vi "9219-9237_3-2.vi"() -> ()   [LabVIEW 2013]
uses:
  <vilib>/Analysis/baseanly.llb/Mean (DBL).vi
  <vilib>/DAQmx/read.llb/DAQmx Read (Analog 1D Wfm NChan NSamp).vi
  <vilib>/measure/mascope.llb/Amplitude and Levels 1 chan.vi
  <vilib>/measure/mamon.llb/Trigger Detection for 1 Channel.vi
  <vilib>/Waveform/WDTOps.llb/WDT Append Waveforms DBL.vi
  <vilib>/DAQmx/miscellaneous.llb/DAQmx Fill In Error Info.vi
  <vilib>/measure/NI_MAPro.lvlib
  <vilib>/measure/mascope.llb/Pulse Measurements 1 chan.vi
  <vilib>/Analysis/NI_AALBase.lvlib
panel:
  in  "탭 컨트롤":T1(tab)
  in  "Force cal val":bool
  out "diff 4":dbl
  out "diff 3":dbl
  out "diff 2":dbl
  out "B 2-4":dbl(slide)
  out "B 1-3":dbl(slide)
  out "Balance 2/4":dbl format="%#_3g"
  out "Balance 1/3":dbl format="%#_3f"
  out "Triggered Force graph":waveform(dbl)(graph)
  out "bonding force":dbl caption="Bonding force (kg)" format="%0.2f"
  out "vaccum":waveform(dbl)(graph)
  out "Bondtime":dbl caption="Bonding time" format="%.3f"
  out "vacum":dbl format="%#_3f"
  out "trigger location":dbl caption="트리거 rising" format="%#.3f"
  out "trigger location 2":dbl caption="트리거 falling" format="%#.3f"
  out "level1 4":dbl caption="right F" format="%.2g"
  out "level1 3":dbl caption="rear F" format="%.2g"
  out "level1 2":dbl caption="left F" format="%.2g"
  out "level1":dbl caption="front F" format="%.2g"
  out "diff 1":dbl
  out "vaccum 차트 3":waveform(dbl)(graph)
  out "Force raw chart":waveform(dbl)[](graph)
  out "x-y 2":u32
  out "x-y":u32
  out "Filtered force 차트":waveform(dbl)[](graph)
  out "Force raw graph":waveform(dbl)[](graph)
  out "Filtered force 그래프":waveform(dbl)[](graph)
  in  "display":bool
  out "Strain front":dbl(graph)
  out "Strain left":dbl(graph)
  out "Strain rear":dbl(graph)
  out "Strain right":dbl(graph)
  out "data":dynamicdata(graph) caption="데이터"
  in  "reference levels":T2={"high ref level"=90.0, "mid ref level"=50.0, "low ref level"=10.0, "ref units"=1} caption="참조 레벨" {"ref units" items=["절대적인", "퍼센트"]; "high ref level" format="%0.2f"; "low ref level" format="%0.2f"; "mid ref level" format="%0.2f"}
  in  "percent level settings":T3={"method"=enum."auto select", "histogram size"=256, "histogram method"=enum."mode", "reserved"=1.0} caption="퍼센트 레벨 셋팅" {"reserved" format="%0.2f"}
  in  "bonding time trigger edge level":dbl=0.2 format="%#_13g"
  out "front mean":dbl format="%0.2f"
  out "left mean":dbl format="%0.2f"
  out "rear mean 3":dbl format="%0.2f"
  out "right mean 4":dbl format="%0.2f"
  in  "Force trigger minimum level":dbl=0.5 format="%#_13g"
  out "force offset":dbl
  in  "정지":bool
  # "Die Attach Machine Monitoring"
  # "1> 앞쪽 힘이 큰 경우\n1< 뒷쪽 힘이 큰 경우"
  # "1> 왼쪽 힘이 큰 경우\n1< 오른쪽 힘이 큰 경우"
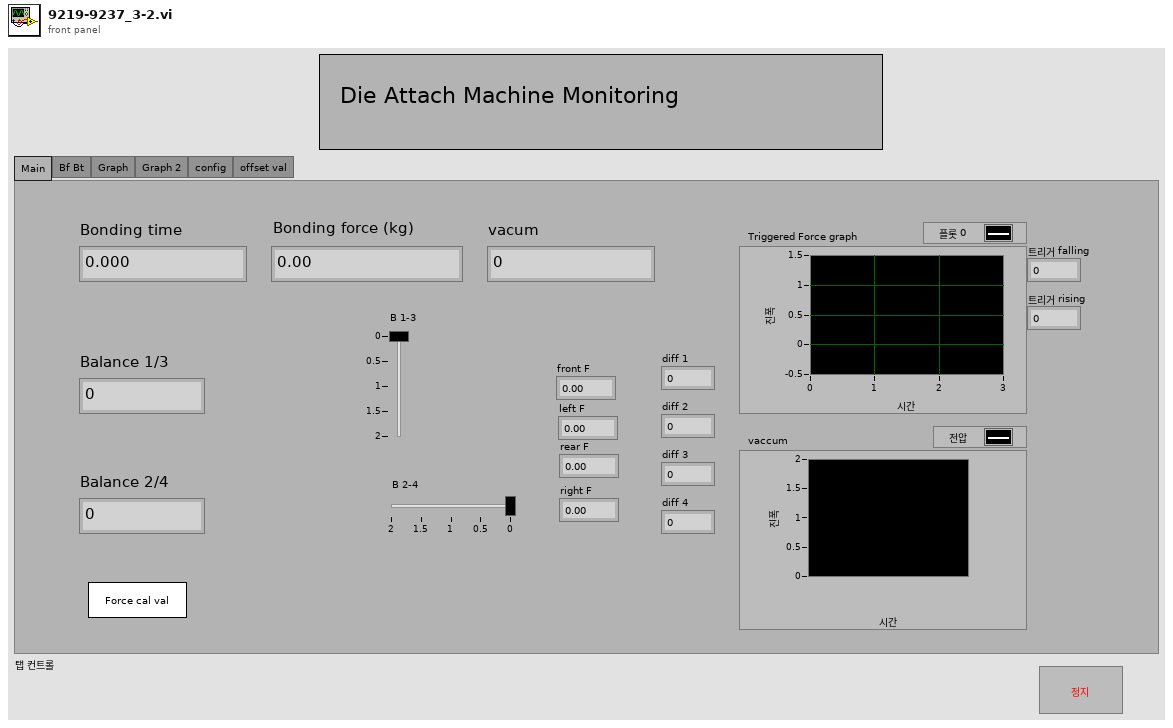
[diagram p1: front panel]
types:
  T1 = enum32{"Main", "Bf Bt", "Graph", "Graph 2", "config", "offset val"}
  T2 = cluster{"high ref level":dbl, "mid ref level":dbl, "low ref level":dbl, "ref units":u16}
  T3 = cluster{"method":enum32{"histogram", "peak", "auto select"}, "histogram size":i32, "histogram method":enum16{"mode"}, "reserved":dbl}
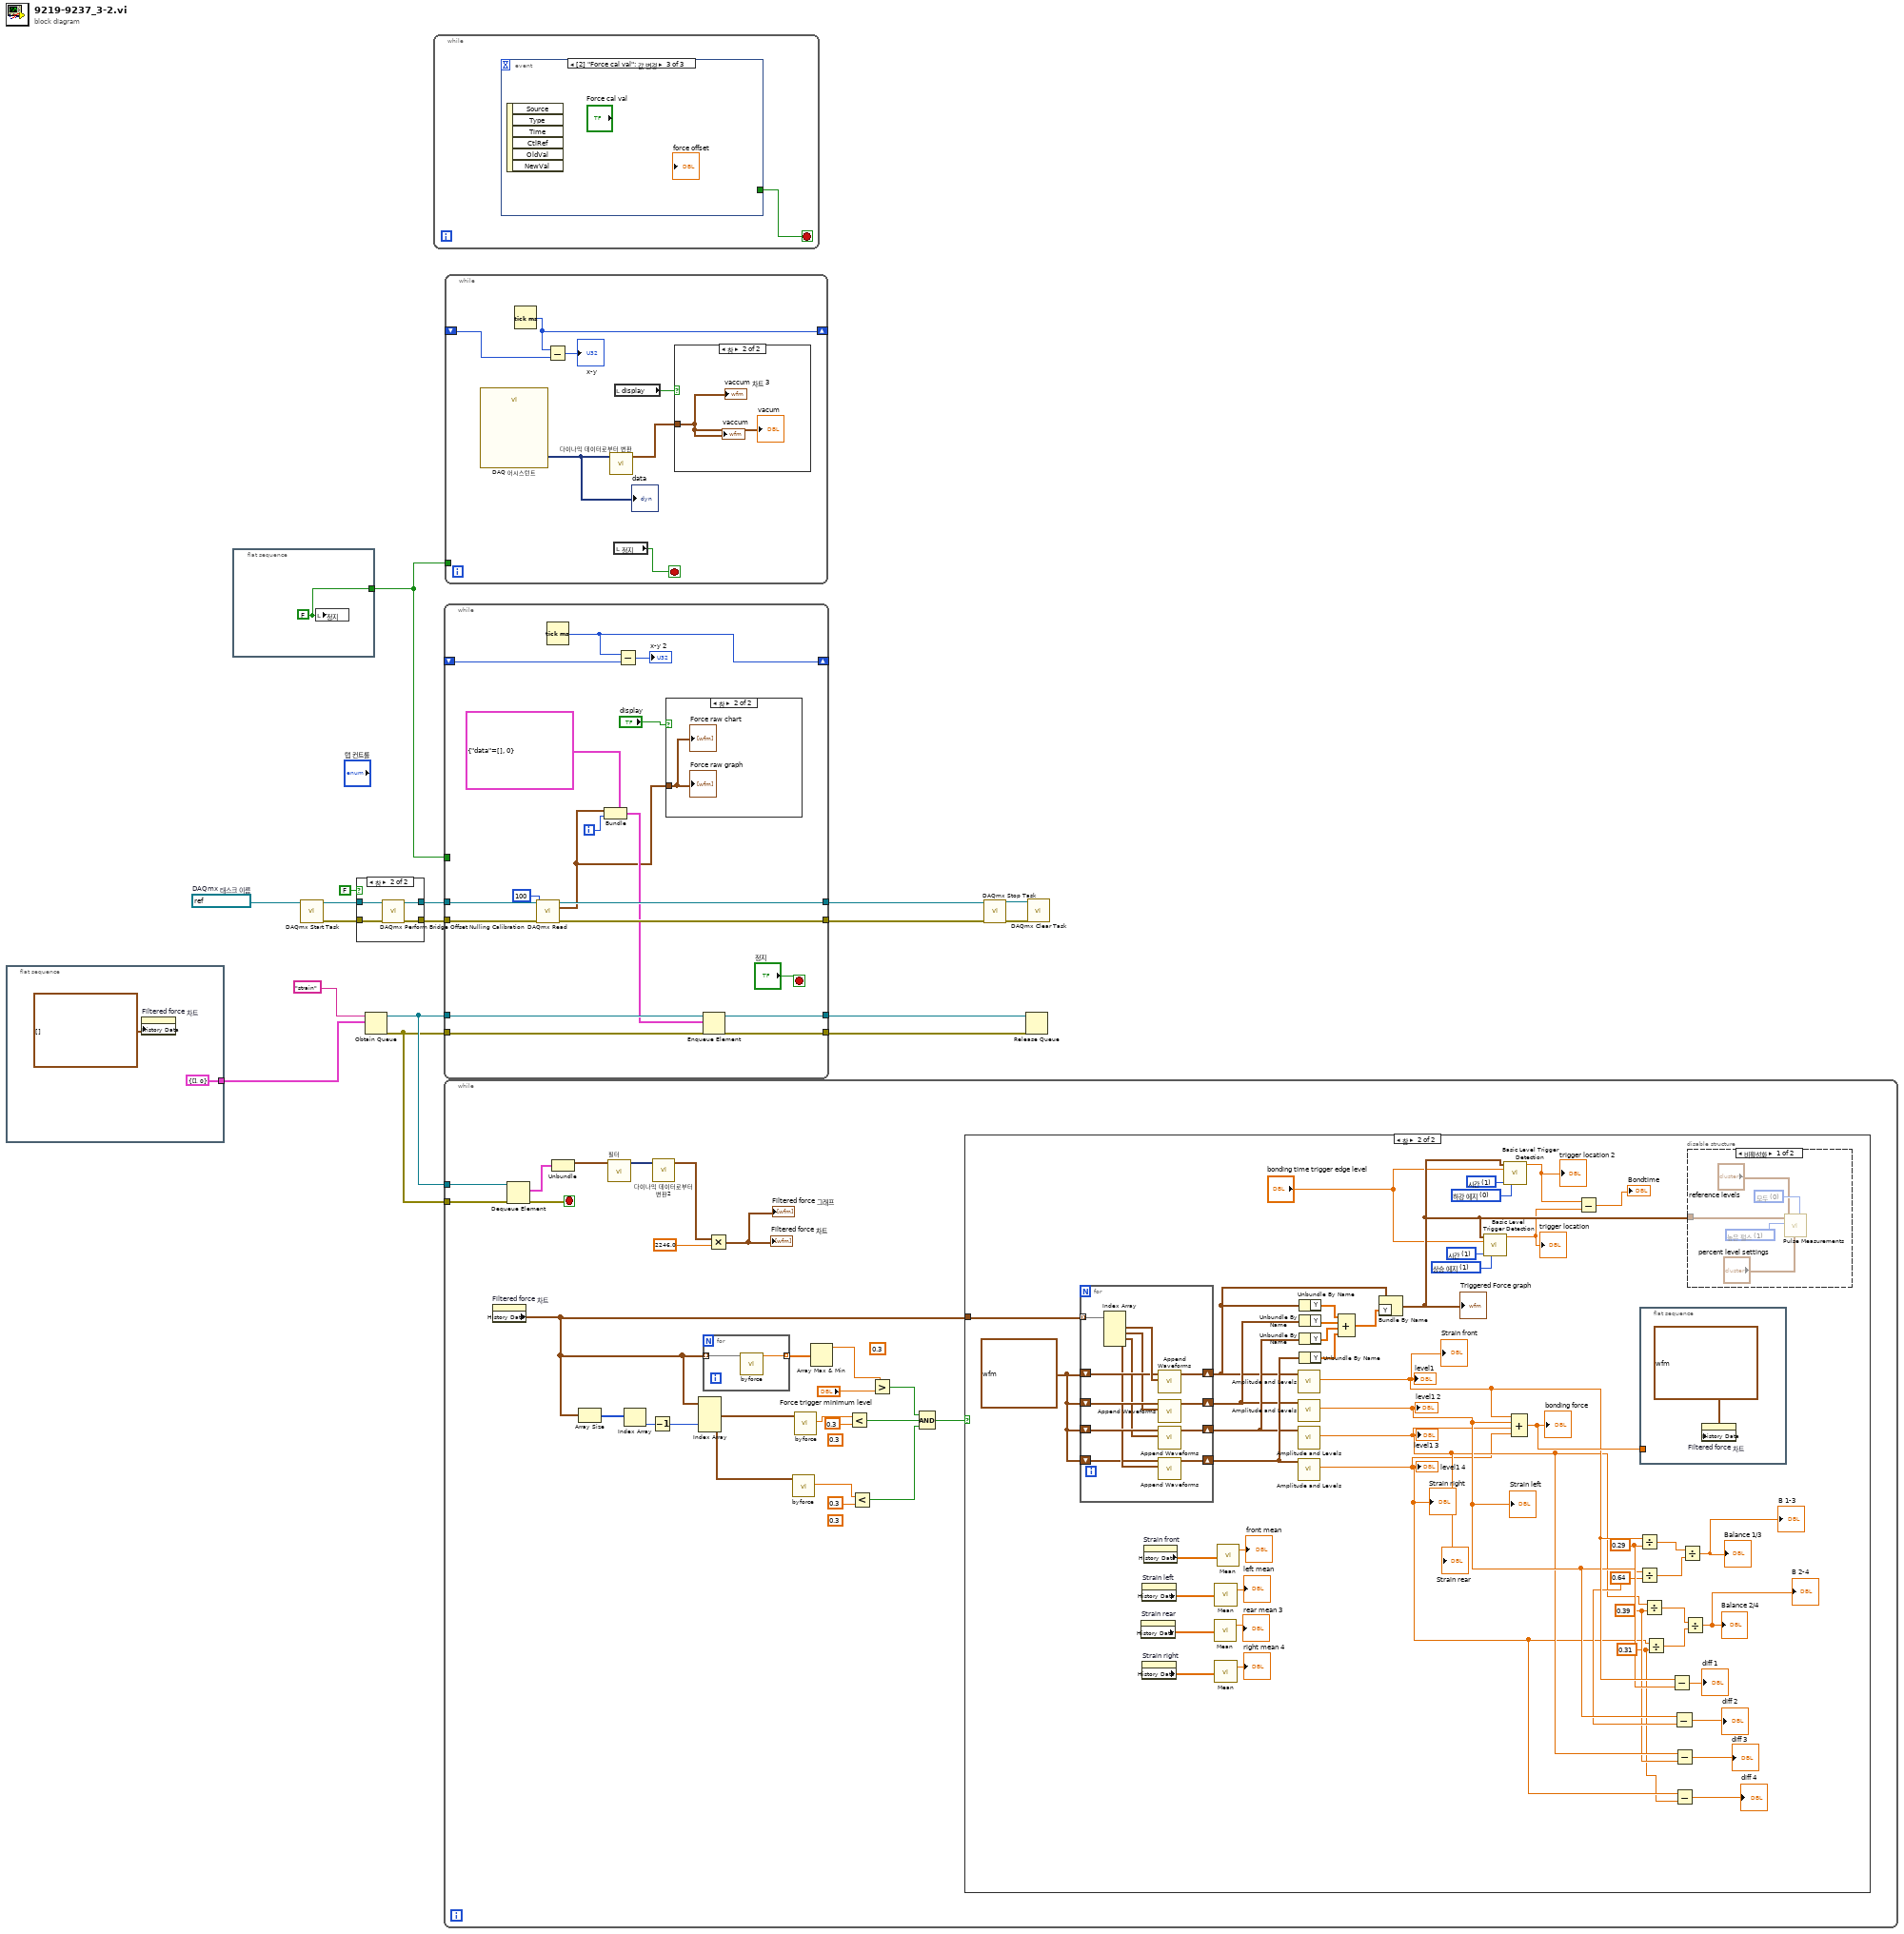
[diagram p0: block diagram]
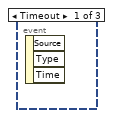
[diagram p3: hidden frame]
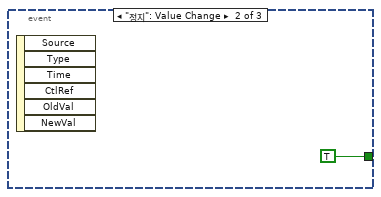
[diagram p4: hidden frame]
diagram:
  w15 = refnum<k21> "9237_task"  # DAQmx 태스크 이름
  n1 = flat-sequence {
    tunnel: [cluster{"data":waveform(dbl)[], i32} {"data"=[], 0}] -> w6
    frame #0 {
      n2 = property on="Filtered force 차트" class="WFChart (엄격한)"("History Data"=waveform(dbl)[][] [] ("히스토리 데이터")) -> ()  [unwired: 2 in, 2 out]
    }
  }
  n3 = flat-sequence {
    tunnel: [w20] -> w12
    frame #0 {
      w20 = FALSE ("정지")
      n4 = local write "정지"(w20) -> ()
    }
  }
  n5 = call <vilib>:"DAQmx Start Task.vi"("task/channels in"=w15) -> ("task out"=w5:refnum<k21>, "error out"=w4:errorcluster)  [unwired: 13 in]
  n6 = case shown="참" FALSE {
    tunnel: w5 -> [w22 w26]
    tunnel: w4 -> [w21 w25]
    tunnel: [w21 w24] -> w3
    tunnel: [w22 w23] -> w2
    frame False {
    }
    frame True {
      n7 = call <vilib>:"DAQmx Perform Bridge Offset Nulling Calibration.vi"("task/channels in"=w26, "error in"=w25) -> ("task out"=w23:refnum<k21>, "error out"=w24:errorcluster)  [unwired: 12 in]
    }
  }
  n8 = Obtain Queue(name (unnamed)="strain" ("이름(이름없음)"), element data type=w6) -> (queue out=w10:refnum<queue>, error out=w8:errorcluster)  [unwired: 3 in, 1 out]
  n9 = while {
    stop <- w27 stop-if-true
    n10 = event shown="[2] \"Force cal val\": 값 변경" {
      selector: _ -> [_ _ _]
      dyn-events: _ -> [_ _ _]
      timeout: _ -> [_ _ _]
      tunnel: [_ TRUE _] -> w27
      event Timeout {
        n11 = event-data() -> ()  [unwired: 1 in, 3 out]
      }
      event "정지": Value Change {
        n12 = event-data() -> ()  [unwired: 1 in, 6 out]
      }
      event "Force cal val": Value Change {
        n13 = event-data() -> ()  [unwired: 1 in, 6 out]
      }
    }
  }
  n14 = while {
    tunnel: w3 -> [w46]
    tunnel: w2 -> [w45]
    tunnel: [w44] -> w17
    tunnel: [w43] -> w16
    tunnel: w12 -> [_]
    tunnel: w10 -> [w40]
    tunnel: [w39] -> w9
    tunnel: w8 -> [w38]
    tunnel: [w37] -> w7
    shift-right: [w32] -> _
    shift-left: _ -> [w33]
    i -> [w35]
    stop <- "정지" stop-if-true
    n15 = call-poly <vilib>:"DAQmx Read.vi"("task/channels in"=w45, "number of samples per channel"=100, "error in"=w46) -> ("task out"=w43:refnum<k21>, "data"=w30:waveform(dbl)[], "error out"=w44:errorcluster)  [unwired: 10 in]
    n16 = Tick Count (ms)() -> (millisecond timer value=w32:u32)
    n17 = Bundle(cluster=cluster{"data":waveform(dbl)[], i32} {"data"=[], 0}, "data"=w30, w35) -> (w34:cluster{"data":waveform(dbl)[], i32})
    n18 = Subtract(x=w32, y=w33) -> (x-y=→"x-y 2":u32)
    n19 = case shown="참" "display" {
      tunnel: w30 -> [_ w47]
      frame False {
      }
      frame True {
        "Force raw graph" <- w47
        "Force raw chart" <- w47
      }
    }
    n20 = Enqueue Element(queue=w40, element=w34, error in (no error)=w38) -> (queue out=w39:refnum<queue>, error out=w37:errorcluster)  [unwired: 1 in, 1 out]
  }
  n21 = while {
    tunnel: w10 -> [w73]
    tunnel: w8 -> [w72]
    stop <- w71 stop-if-true
    (unwired) 0.3 ("y")
    (unwired) 0.3 ("y")
    (unwired) 0.3 ("y")
    n22 = property on="Filtered force 차트" class="WFChart (엄격한)"() -> ("History Data"=w55:waveform(dbl)[][])  [unwired: 2 in, 2 out]
    n23 = Dequeue Element(queue=w73, error in (no error)=w72) -> (element=w69:cluster{"data":waveform(dbl)[], i32}, error out=w71:errorcluster)  [unwired: 1 in, 2 out]
    n24 = Unbundle(w69) -> ("data"=w54:waveform(dbl)[])  [unwired: 1 out]
    n25 = Array Size(array=w55) -> (size(s)=w68:i32[])
    n26 = call "필터"("Signal"=w54) -> ("Filtered Signal"=w53:dynamicdata)  [unwired: 9 in, 1 out]
    n27 = Index Array(array=w68) -> (element=w67:i32)  [unwired: 1 in]
    n28 = Decrement(x=w67) -> (x-1=w66:i32)
    n29 = call "다이나믹 데이터로부터 변환2"("Dynamic Data Type"=w53) -> ("Array of Waveform"=w52:waveform(dbl)[])  [unwired: 3 in]
    n30 = Index Array(array=w55, index (row) #2=w66) -> (element #1=w65:waveform(dbl)[], element #2=w64:waveform(dbl)[])  [unwired: 3 in]
    n31 = for {
      tunnel: w55 -> [w141] mode=indexing
      tunnel: [w140] -> w61 mode=indexing
      n32 = call "byforce.vi"("History Data"=w141) -> ("mean"=w140:dbl)  [unwired: 8 in, 2 out]
    }
    n33 = Multiply(x=w52, y=2246.0) -> (x*y=→"Filtered force 그래프" →"Filtered force 차트":waveform(dbl)[])
    n34 = call "byforce.vi"("History Data"=w64) -> ("max"=w49:dbl)  [unwired: 8 in, 2 out]
    n35 = call "byforce.vi"("History Data"=w65) -> ("max"=w50:dbl)  [unwired: 8 in, 2 out]
    n36 = Array Max & Min(array=w61) -> (max value=w60:dbl)  [unwired: 3 out]
    n37 = Less?(x=w50, y=0.3) -> (x < y?=w58:bool)
    n38 = Less?(x=w49, y=0.3) -> (x < y?=w57:bool)
    n39 = Greater?(x=w60, y="Force trigger minimum level") -> (0:w59:bool)
    n40 = Compound Arithmetic op=AND(w59, w58, w57) -> (w56:bool)
    n41 = case shown="참" w56 {
      tunnel: w55 -> [_ w120]
      frame False {
      }
      frame True {
        w100 = u16 1 items=["인덱스", "시간"] ("location mode")
        w99 = u16 0 items=["하강 에지", "상승 에지"] ("trigger slope")
        w101 = u16 1 items=["인덱스", "시간"] ("location mode")
        w102 = u16 1 items=["하강 에지", "상승 에지"] ("trigger slope")
        w87 = 0.31 ("y")
        w89 = 0.39 ("y")
        w91 = 0.64 ("y")
        w93 = 0.29 ("y")
        w119 = waveform(dbl) {"t0"=timestamp(0 s since 1904-01-01), "dt"=0.00062, "Y"=[]} ("원소")
        n42 = for {
          tunnel: w120 -> [w139] mode=indexing
          shift-right: [w138] -> w110
          shift-left: w119 -> [w133]
          shift-right: [w137] -> w111
          shift-left: w119 -> [w132]
          shift-right: [w136] -> w112
          shift-left: w119 -> [w130]
          shift-right: [w135] -> w113
          shift-left: w119 -> [w127]
          n43 = Index Array(array=w139) -> (element #1=w134:waveform(dbl), element #2=w131:waveform(dbl), element #3=w129:waveform(dbl), element #4=w128:waveform(dbl))  [unwired: 4 in]
          n44 = call-poly <vilib>:"Append Waveforms.vi"("waveform B"=w134, "waveform A"=w133) -> ("waveform out"=w138:waveform(dbl))  [unwired: 8 in, 1 out]
          n45 = call-poly <vilib>:"Append Waveforms.vi"("waveform B"=w131, "waveform A"=w132) -> ("waveform out"=w137:waveform(dbl))  [unwired: 8 in, 1 out]
          n46 = call-poly <vilib>:"Append Waveforms.vi"("waveform B"=w129, "waveform A"=w130) -> ("waveform out"=w136:waveform(dbl))  [unwired: 8 in, 1 out]
          n47 = call-poly <vilib>:"Append Waveforms.vi"("waveform B"=w128, "waveform A"=w127) -> ("waveform out"=w135:waveform(dbl))  [unwired: 8 in, 1 out]
        }
        n48 = property on="Strain rear" class="WFChart (엄격한)"() -> ("History Data"=w79:dbl[])  [unwired: 2 in, 2 out]
        n49 = property on="Strain left" class="WFChart (엄격한)"() -> ("History Data"=w78:dbl[])  [unwired: 2 in, 2 out]
        n50 = property on="Strain right" class="WFChart (엄격한)"() -> ("History Data"=w80:dbl[])  [unwired: 2 in, 2 out]
        n51 = property on="Strain front" class="WFChart (엄격한)"() -> ("History Data"=w81:dbl[])  [unwired: 2 in, 2 out]
        n52 = call-poly <vilib>:"Mean.vi"("X"=w79) -> ("mean"=→"rear mean 3":dbl)  [unwired: 1 out]
        n53 = call-poly <vilib>:"Mean.vi"("X"=w78) -> ("mean"=→"left mean":dbl)  [unwired: 1 out]
        n54 = call-poly <vilib>:"Mean.vi"("X"=w80) -> ("mean"=→"right mean 4":dbl)  [unwired: 1 out]
        n55 = call-poly <vilib>:"Mean.vi"("X"=w81) -> ("mean"=→"front mean":dbl)  [unwired: 1 out]
        n56 = call-poly <vilib>:"Amplitude and Levels.vi"("signal in"=w110) -> ("high state level"=w94:dbl)  [unwired: 7 in, 3 out]
        "level1" <- w94
        "Strain front" <- w94
        n57 = call-poly <vilib>:"Amplitude and Levels.vi"("signal in"=w111) -> ("high state level"=w92:dbl)  [unwired: 7 in, 3 out]
        "level1 2" <- w92
        "Strain left" <- w92
        n58 = call-poly <vilib>:"Amplitude and Levels.vi"("signal in"=w112) -> ("high state level"=w90:dbl)  [unwired: 7 in, 3 out]
        "level1 3" <- w90
        "Strain rear" <- w90
        n59 = call-poly <vilib>:"Amplitude and Levels.vi"("signal in"=w113) -> ("high state level"=w88:dbl)  [unwired: 7 in, 3 out]
        "level1 4" <- w88
        "Strain right" <- w88
        n60 = Unbundle By Name(w110) -> ("Y"=w115:dbl[])
        n61 = Unbundle By Name(w111) -> ("Y"=w116:dbl[])
        n62 = Unbundle By Name(w112) -> ("Y"=w117:dbl[])
        n63 = Unbundle By Name(w113) -> ("Y"=w118:dbl[])
        n64 = Compound Arithmetic op=ADD(w115, w116, w117, w118) -> (w114:dbl[])
        n65 = Bundle By Name(cluster=w110, "Y"=w114) -> (w98:waveform(dbl))
        "Triggered Force graph" <- w98
        n66 = call-poly <vilib>:"Basic Level Trigger Detection.vi"("signal in"=w98, "level"="bonding time trigger edge level", "location mode"=w101, "trigger slope"=w102) -> ("trigger location"=w96:dbl)  [unwired: 9 in, 2 out]
        "trigger location" <- w96
        n67 = call-poly <vilib>:"Basic Level Trigger Detection.vi"("signal in"=w98, "level"="bonding time trigger edge level", "location mode"=w100, "trigger slope"=w99) -> ("trigger location"=w97:dbl)  [unwired: 9 in, 2 out]
        "trigger location 2" <- w97
        n68 = Compound Arithmetic op=ADD(w94, w92, w90, w88) -> (w109:dbl)
        "bonding force" <- w109
        n69 = Subtract(x=w97, y=w96) -> (x-y=→"Bondtime":dbl)
        n70 = Divide(x=w94, y=w93) -> (x/y=w108:dbl)
        n71 = Divide(x=w92, y=w91) -> (x/y=w107:dbl)
        n72 = flat-sequence {
          tunnel: w109 -> [_]
          frame #0 {
            n73 = property on="Filtered force 차트" class="WFChart (엄격한)"("History Data"=waveform(dbl)[][] [[{"t0"=timestamp(0 s since 1904-01-01), "dt"=0.00062, "Y"=[]}]] ("히스토리 데이터")) -> ()  [unwired: 2 in, 2 out]
          }
        }
        n74 = Divide(x=w90, y=w89) -> (x/y=w105:dbl)
        n75 = Divide(x=w88, y=w87) -> (x/y=w106:dbl)
        n76 = Subtract(x=w94, y=w93) -> (x-y=→"diff 1":dbl)
        n77 = Subtract(x=w92, y=w91) -> (x-y=→"diff 2":dbl)
        n78 = Subtract(x=w90, y=w89) -> (x-y=→"diff 3":dbl)
        n79 = Subtract(x=w88, y=w87) -> (x-y=→"diff 4":dbl)
        n80 = Divide(x=w108, y=w107) -> (x/y=→"Balance 1/3" →"B 1-3":dbl)
        n81 = Divide(x=w105, y=w106) -> (x/y=→"Balance 2/4" →"B 2-4":dbl)
        n82 = disable-structure shown="비활성화" {
          disable-tunnel: w98 -> [w121 _]
          frame Disabled {
            w124 = u16 1 items=["낮은 펄스", "높은 펄스"] ("polarity (high)")
            w125 = u16 0 items=["모두", "주기 및 주기 점유율 없음"] ("export mode")
            n83 = call-poly <vilib>:"Pulse Measurements.vi"("export mode"=w125, "percent level settings"="percent level settings", "reference levels"="reference levels", "polarity (high)"=w124, "signal in"=w121) -> ()  [unwired: 2 in, 5 out]
          }
          frame Enabled {
          }
        }
      }
    }
  }
  n84 = while {
    tunnel: w12 -> [_]
    shift-right: [w147] -> _
    shift-left: _ -> [w146]
    stop <- w148 stop-if-true
    n85 = call "DAQ 어시스턴트"() -> ("data"=w144:dynamicdata)  [unwired: 16 in, 3 out]
    "data" <- w144
    n86 = Tick Count (ms)() -> (millisecond timer value=w147:u32)
    n87 = Subtract(x=w147, y=w146) -> (x-y=→"x-y":u32)
    n88 = call "다이나믹 데이터로부터 변환"("Dynamic Data Type"=w144) -> ("Waveform"=w143:waveform(dbl))  [unwired: 3 in]
    n89 = local read "정지"() -> (w148:bool)
    n90 = local read "display"() -> (w142:bool)
    n91 = case shown="참" w142 {
      tunnel: w143 -> [_ w149]
      frame False {
      }
      frame True {
        "vaccum" <- w149
        "vaccum 차트 3" <- w149
        "vacum" <- w149
      }
    }
  }
  n92 = call <vilib>:"DAQmx Stop Task.vi"("task/channels in"=w16, "error in"=w17) -> ("task out"=w13:refnum<k21>, "error out"=w14:errorcluster)  [unwired: 12 in]
  n93 = Release Queue(queue=w9, error in (no error)=w7) -> ()  [unwired: 1 in, 3 out]
  n94 = call <vilib>:"DAQmx Clear Task.vi"("task in"=w13, "error in"=w14) -> ()  [unwired: 13 in, 1 out]
